vi "Test_TerminalBinding_ValueOK.vi"(8 "error in (no error)":errorcluster, 11 "TestCase in":refnum<class "TestTransport.lvclass">) -> (0 "error out":errorcluster, 3 "TestCase out":refnum<class "TestTransport.lvclass">)   [LabVIEW 2017, in "Transport.lvlib" / "TestTransport.lvclass"]
uses:
  TestTransport.lvclass
  TerminalBinding/TerminalBinding.lvclass
panel:
  out "An I32 Terminal":i32
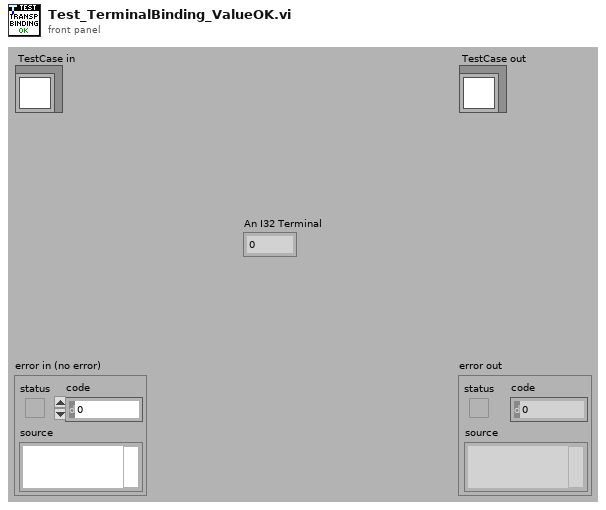
[diagram p1: front panel]
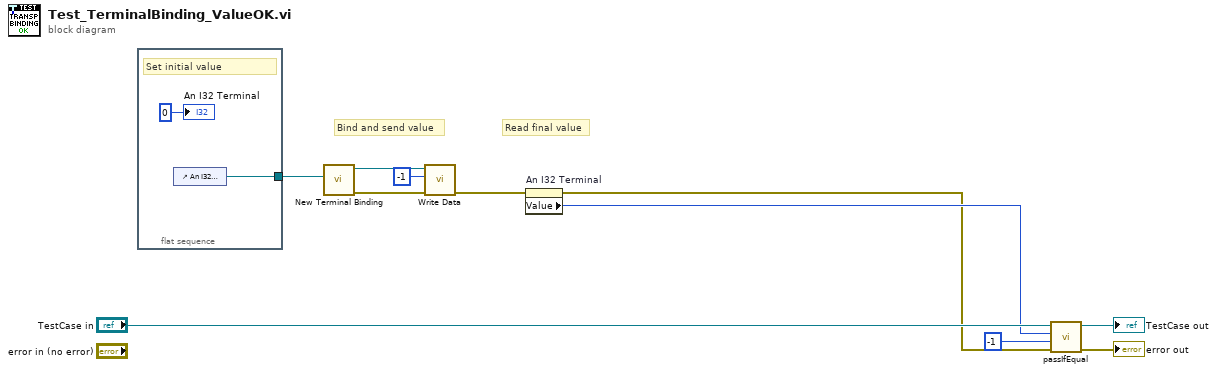
[diagram p0: block diagram]
diagram:
  # "Bind and send value"
  # "Read final value"
  n1 = flat-sequence {
    tunnel: [w12] -> w3
    frame #0 {
      # "Set initial value"
      n2 = control-ref of="An I32 Terminal"() -> (w12:refnum<vi>)
      "An I32 Terminal" <- 0 ("An I32 Terminal")
    }
  }
  n3 = call "New Terminal Binding.vi"("Ctl Refnum"=w3) -> ("error out"=w2:errorcluster, "TerminalBinding"=w6:refnum<class "TerminalBinding.lvclass">)  [unwired: 9 in]
  n4 = call-dynamic "Write Data.vi"("error in (no error)"=w2, "Value"=-1, "TerminalBinding in"=w6) -> ("error out"=w4:errorcluster)  [unwired: 7 in, 1 out]
  n5 = property on="An I32 Terminal" class="DigNum (strict)"(error in=w4) -> (error out=w1:errorcluster, "Value"=w7:i32)  [unwired: 1 in, 1 out]
  n6 = call-dynamic "passIfEqual.vi"("error in (no error)"=w1, "y"=-1, "x"=w7, "TestCase in"="TestCase in") -> ("error out"=→"error out":errorcluster, "TestCase out"=→"TestCase out":refnum<class "TestTransport.lvclass">)  [unwired: 6 in]
